vi "plot.vi"(10 "angle":dbl(slide) scale=0.0..360.0, 11 "speed":dbl(slide) scale=0.0..1.0) -> (3 "XY Graph":cluster{"Array":dbl[], "Array 2":dbl[]}[](graph))   [LabVIEW 2018]
panel:
  out "y":dbl
  out "x":dbl
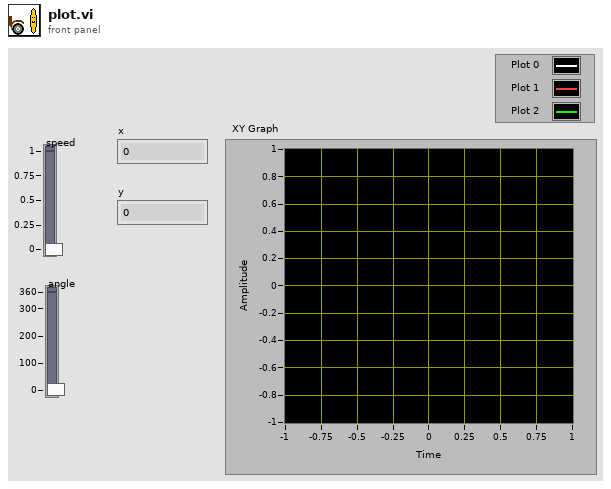
[diagram p1: front panel]
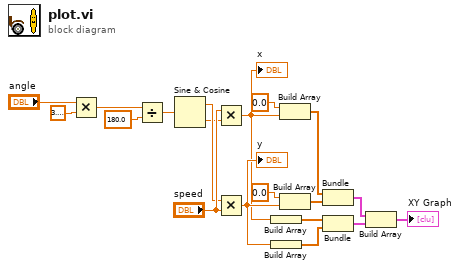
[diagram p0: block diagram]
diagram:
  n1 = Multiply(x="angle", y=3.141592653589793) -> (x*y=w14:dbl)
  n2 = Divide(x=w14, y=180.0) -> (x/y=w12:dbl)
  n3 = Sine & Cosine(0:w12) -> (1:w2:dbl, 2:w1:dbl)
  n4 = Multiply(x="speed", y=w1) -> (x*y=w8:dbl)
  "x" <- w8
  n5 = Multiply(x=w2, y="speed") -> (x*y=w9:dbl)
  "y" <- w9
  n6 = Build Array(w8) -> (w4:dbl[])
  n7 = Build Array(w9) -> (w3:dbl[])
  n8 = Build Array(0.0 ("element"), w8) -> (w10:dbl[])
  n9 = Build Array(0.0 ("element"), w9) -> (w5:dbl[])
  n10 = Bundle(w10, w5) -> (w19:cluster{dbl[], dbl[]})  [unwired: 1 in]
  n11 = Bundle(w4, w3) -> (w17:cluster{dbl[], dbl[]})  [unwired: 1 in]
  n12 = Build Array(w19, w17) -> (→"XY Graph":cluster{dbl[], dbl[]}[])
